vi "Close File.vi"(8 "error in (no error)":errorcluster, 11 "TXT in":refnum<class "TXT.lvclass">) -> (0 "error out":errorcluster)   [LabVIEW 2017, in "TXT.lvlib" / "TXT.lvclass"]
uses:
  TXT.lvclass
  TXT.lvclass/TXT.ctl
  Public/Documents/National Instruments/NI VeriStand 2017/Custom Devices/Shared Variables CD 2.0/Data/ImportExport.lvlibp/ConfigFile/ConfigFile.lvclass
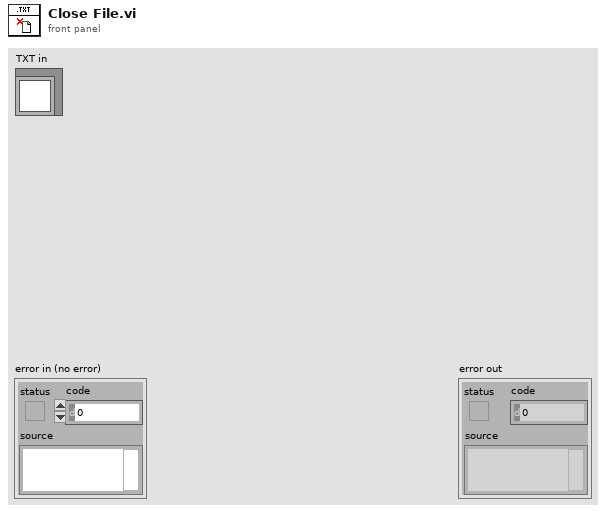
[diagram p1: front panel]
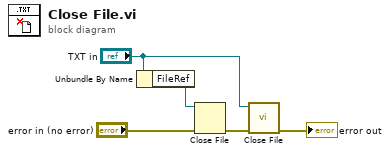
[diagram p0: block diagram]
diagram:
  n1 = Unbundle By Name("TXT in") -> ("FileRef"=w1:refnum<file>)
  n2 = Close File(refnum=w1, error in="error in (no error)") -> (error out=w3:errorcluster)  [unwired: 1 out]
  n3 = call-parent "Close File.vi"("error in (no error)"=w3, "ConfigFile in"="TXT in") -> ("error out"=→"error out":errorcluster)  [unwired: 9 in]
